vi "Run Test.vi"(8 "error in (no error)":errorcluster, 11 "Test Class in":refnum<class "Test Class.lvclass">) -> (0 "error out":errorcluster, 1 "Positions":i32[](array[numeric]), 2 "Tests Passed":bool[](array[boolean]), 3 "Test Class out":refnum<class "Test Class.lvclass">, 5 "Fail Codes":string[](array[string]))   [LabVIEW 2017, in "Test Class.lvclass"]
uses:
  Test Class.lvclass
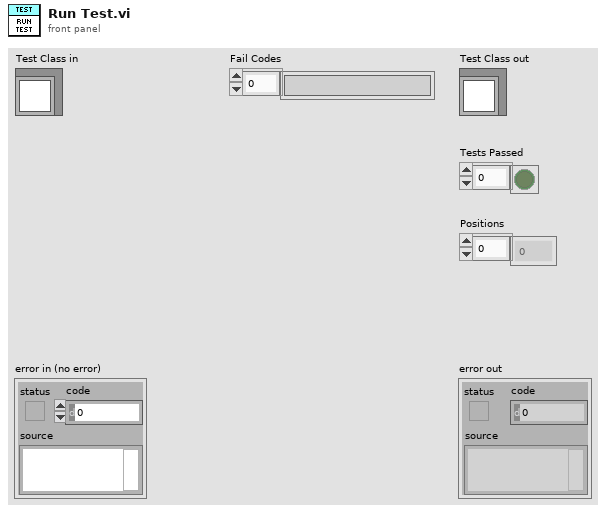
[diagram p1: front panel]
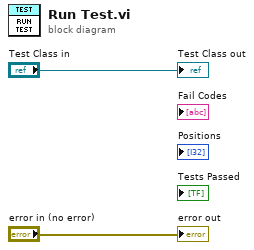
[diagram p0: block diagram]
diagram:
  "error out" <- "error in (no error)"
  "Test Class out" <- "Test Class in"
